vi "Cast Object to Variant.vi"(8 "error in (no error)":errorcluster, 9 "datatype and defaults":variant, 11 "JSON Object in":refnum<class "JSON Object.lvclass">) -> (0 "error out":errorcluster, 2 "Variant":variant)   [LabVIEW 2015, in "LVJSON.lvlib" / "JSON Object.lvclass"]
uses:
  JSON Object.lvclass
  Get Value (Numeric Value).vi
  Get Value (Boolean Value).vi
  Get Value (Object).vi
  Get Value (Array).vi
  Get Value (String Value).vi
  <vilib>/Utility/Data Type/NI_Data Type.lvlib
  LVJSON.lvlib
  JSON Array/JSON Array.lvclass
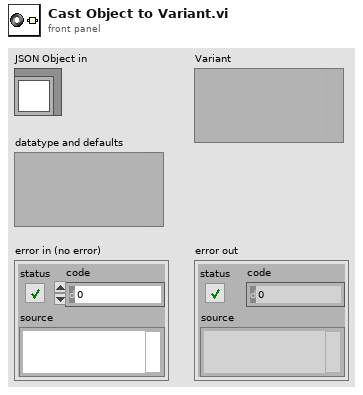
[diagram p1: front panel]
types:
  T1 = typedef "NI_Data Type.lvlib/Data Type.ctl" = enum8{"Invalid Type", "Void", "I8", "I16", "I32", "I64", "U8", "U16", "U32", "U64", "Single Float", "Double Float", "Extended Float", "Single Complex", "Double Complex", "Extended Complex", "Enum U8", "Enum U16", "Enum U32", "Enum U64", "Single Float With Unit", "Double Float With Unit", "Extended Float With Unit", "Single Complex with Unit", "Double Complex with Unit", "Extended Complex with Unit", "Boolean", "String", "Path", "Picture", "Tag", "Array", "Cluster", "Variant", "LV Variant", "Waveform", "Timestamp", "Digital Waveform", "Digital Data", "ExpressData", "Refnum", "External Data", "VI", "Poly VI", "LabVIEW Class Instance", "Fixed Point"}
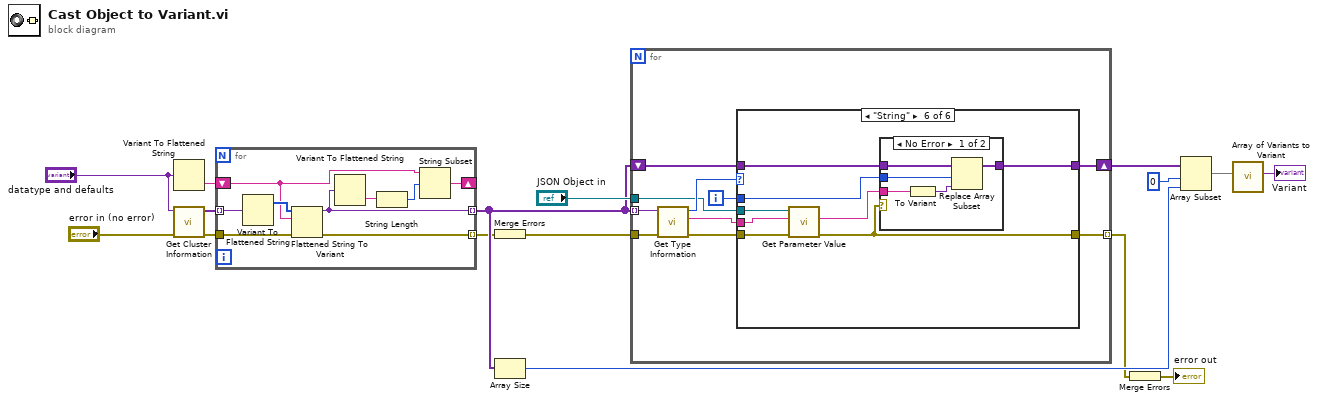
[diagram p0: block diagram]
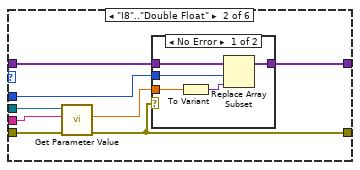
[diagram p3: hidden frame]
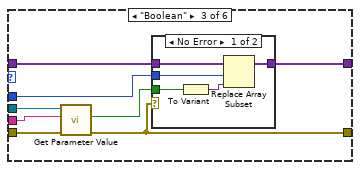
[diagram p5: hidden frame]
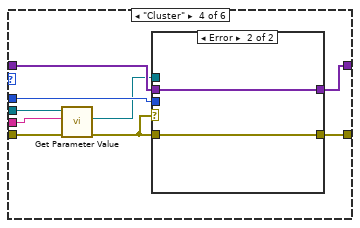
[diagram p7: hidden frame]
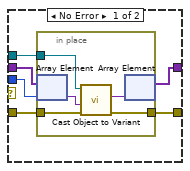
[diagram p8: hidden frame]
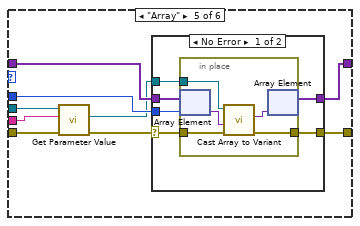
[diagram p9: hidden frame]
diagram:
  n1 = Variant To Flattened String(Variant="datatype and defaults") -> (data string=w8:string)  [unwired: 1 out]
  n2 = call <vilib>:"Get Cluster Information.vi"("error in (no error)"="error in (no error)", "Variant"="datatype and defaults") -> ("error out"=w6:errorcluster, "Cluster Elements"=w7:variant[])  [unwired: 8 in]
  n3 = for {
    tunnel: w7 -> [w25] mode=indexing
    tunnel: [w23] -> w3 mode=indexing
    shift-right: [w19] -> _
    shift-left: w8 -> [w22]
    tunnel: w6 -> [w18]
    tunnel: [w17] -> w1 mode=indexing
    n4 = Variant To Flattened String(Variant=w25) -> (1:w24:i16[])  [unwired: 1 out]
    n5 = Flattened String To Variant(4:w18, 6:w22, 7:w24) -> (0:w17:errorcluster, 3:w23:variant)
    n6 = Variant To Flattened String(Variant=w23) -> (data string=w21:string)  [unwired: 1 out]
    n7 = String Length(string=w21) -> (length=w20:i32)
    n8 = String Subset(string=w22, offset (0)=w20) -> (substring=w19:string)  [unwired: 1 in]
  }
  n9 = Merge Errors(w1) -> (w2:errorcluster)
  n10 = Array Size(array=w3) -> (size(s)=w13:i32)
  n11 = for {
    tunnel: w3 -> [w35] mode=indexing
    tunnel: "JSON Object in" -> [w32]
    shift-right: [w31] -> w11
    shift-left: w3 -> [w30]
    tunnel: [w28] -> w10 mode=indexing
    tunnel: w2 -> [w26]
    i -> [w29]
    n12 = call <vilib>:"Get Type Information.vi"("error in (no error)"=w26, "Variant"=w35) -> ("error out"=w27:errorcluster, "Name"=w33:string, "Type"=w34:T1)  [unwired: 5 in, 2 out]
    n13 = case shown="\"String\"" w34 {
      tunnel: w33 -> [_ w43 w58 w73 w95 w115]
      tunnel: w32 -> [_ w45 w59 w74 w96 w117]
      tunnel: [w36 w40 w55 w70 w92 w112] -> w31
      tunnel: w30 -> [w36 w42 w57 w72 w94 w114]
      tunnel: w29 -> [_ w41 w56 w71 w93 w113]
      tunnel: [w37 w38 w52 w67 w89 w110] -> w28
      tunnel: w27 -> [w37 w39 w54 w69 w91 w111]
      frame "Invalid Type", Default {
      }
      frame "I8".."Double Float" {
        n14 = call-poly "Get Parameter Value.vi"("error in (no error)"=w39, "key"=w43, "JSON Object in"=w45) -> ("error out"=w38:errorcluster, "value"=w44:dbl)  [unwired: 7 in]
        n15 = case shown="No Error" w38 {
          tunnel: w44 -> [w50 _]
          tunnel: w42 -> [w49 w51]
          tunnel: w41 -> [w48 _]
          tunnel: [w46 w51] -> w40
          frame No Error {
            n16 = To Variant(anything=w50) -> (Variant=w47:variant)
            n17 = Replace Array Subset(array=w49, new element=w47, index=w48) -> (w46:variant[])
          }
          frame Error {
          }
        }
      }
      frame "Boolean" {
        n18 = call-poly "Get Parameter Value.vi"("error in (no error)"=w54, "key"=w58, "JSON Object in"=w59) -> ("error out"=w52:errorcluster, "value"=w53:bool)  [unwired: 7 in]
        n19 = case shown="No Error" w52 {
          tunnel: w53 -> [w64 _]
          tunnel: w57 -> [w63 w65]
          tunnel: w56 -> [w62 _]
          tunnel: [w60 w65] -> w55
          frame No Error {
            n20 = To Variant(anything=w64) -> (Variant=w61:variant)
            n21 = Replace Array Subset(array=w63, new element=w61, index=w62) -> (w60:variant[])
          }
          frame Error {
          }
        }
      }
      frame "Cluster" {
        n22 = call-poly "Get Parameter Value.vi"("error in (no error)"=w69, "key"=w73, "JSON Object in"=w74) -> ("error out"=w66:errorcluster, "value"=w68:refnum<class "JSON Object.lvclass">)  [unwired: 7 in]
        n23 = case shown="Error" w66 {
          tunnel: w68 -> [w80 _]
          tunnel: w72 -> [w79 w87]
          tunnel: w71 -> [w78 _]
          tunnel: [w77 w87] -> w70
          tunnel: w66 -> [w76 w86]
          tunnel: [w75 w86] -> w67
          frame No Error {
            n24 = in-place {
              in-place-border: w80 -> [w85]
              in-place-border: w76 -> [w82]
              in-place-border: [w81] -> w75
              n25 = in-place-array #1(w79, w78) -> (w84:variant)
              n26 = call "Cast Object to Variant.vi"("error in (no error)"=w82, "datatype and defaults"=w84, "JSON Object in"=w85) -> ("error out"=w81:errorcluster, "Variant"=w83:variant)  [unwired: 7 in]
              n27 = in-place-array #1(w83) -> (w77:variant[])  [unwired: 1 out]
            }
          }
          frame Error {
          }
        }
      }
      frame "Array" {
        n28 = call-poly "Get Parameter Value.vi"("error in (no error)"=w91, "key"=w95, "JSON Object in"=w96) -> ("error out"=w88:errorcluster, "value"=w90:refnum<class "JSON Array.lvclass">)  [unwired: 7 in]
        n29 = case shown="No Error" w88 {
          selector: w88 -> [w98 w108]
          tunnel: w90 -> [w102 _]
          tunnel: w94 -> [w101 w109]
          tunnel: w93 -> [w100 _]
          tunnel: [w99 w109] -> w92
          tunnel: [w97 w108] -> w89
          frame No Error {
            n30 = in-place {
              in-place-border: w102 -> [w105]
              in-place-border: w98 -> [w104]
              in-place-border: [w103] -> w97
              n31 = in-place-array #2(w101, w100) -> (w107:variant)
              n32 = call "Cast Array to Variant.vi"("error in (no error)"=w104, "datatype and defaults"=w107, "JSON Array in"=w105) -> ("error out"=w103:errorcluster, "Variant"=w106:variant)  [unwired: 7 in]
              n33 = in-place-array #2(w106) -> (w99:variant[])  [unwired: 1 out]
            }
          }
          frame Error {
          }
        }
      }
      frame "String" {
        n34 = call-poly "Get Parameter Value.vi"("error in (no error)"=w111, "key"=w115, "JSON Object in"=w117) -> ("error out"=w110:errorcluster, "value"=w116:string)  [unwired: 7 in]
        n35 = case shown="No Error" w110 {
          tunnel: w116 -> [w122 _]
          tunnel: w114 -> [w121 w123]
          tunnel: w113 -> [w120 _]
          tunnel: [w118 w123] -> w112
          frame No Error {
            n36 = To Variant(anything=w122) -> (Variant=w119:variant)
            n37 = Replace Array Subset(array=w121, new element=w119, index=w120) -> (w118:variant[])
          }
          frame Error {
          }
        }
      }
    }
  }
  n38 = Merge Errors(w10) -> (→"error out":errorcluster)
  n39 = Array Subset(array=w11, index=0, length=w13) -> (w15:variant[])
  n40 = call "Array of Variants to Variant.vi"("Array"=w15) -> ("Variant"=→"Variant":variant)  [unwired: 10 in]
